vi "getPosition.vi"(6 "Delay between send and receive [ms]":i32=100, 8 "error in (no error)":errorcluster, 11 "Monochromator in":refnum<class "Monochromator.lvclass">) -> (0 "error out":errorcluster, 2 "wavelength":dbl, 3 "Monochromator out":refnum<class "Monochromator.lvclass">)   [LabVIEW 2023, in "horiba.lvlib" / "Monochromator.lvclass"]
doc: "Returns the wavelength value, in nm, of the monochromator's current position."
uses:
  Monochromator.lvclass
  d9b87029-586e-44ee-a6e5-d4a5e0edce38.vi
  b59fd1e7-dcda-425c-bd6c-61aafb79e7f4.vi
  GenericDevice/GenericDevice.lvclass
  WavelengthPosition.ctl
panel:
  # "Connector Pane"
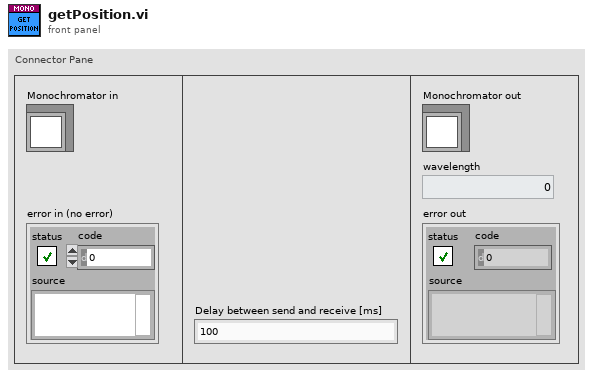
[diagram p1: front panel]
types:
  T1 = typedef "horiba.lvlib/Monochromator.lvclass/WavelengthPosition.ctl" = cluster{"wavelength":dbl}
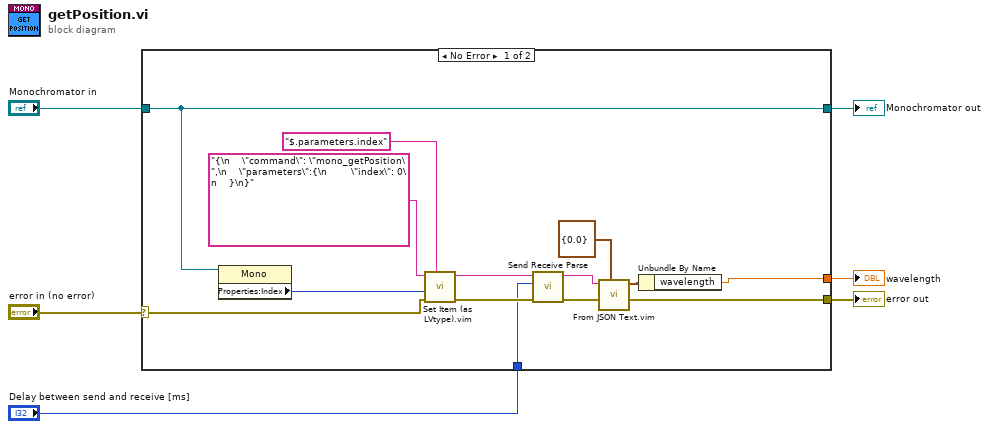
[diagram p0: block diagram]
diagram:
  n1 = case shown="No Error" "error in (no error)" {
    selector: "error in (no error)" -> [w16 w22]
    tunnel: [w15 w22] -> w5
    tunnel: [w18 w21] -> w3
    tunnel: "Monochromator in" -> [w18 w21]
    tunnel: [w8 _] -> w2
    tunnel: "Delay between send and receive [ms]" -> [w7 _]
    frame No Error {
      n2 = property class="Mono"(reference=w18) -> ("Properties:Index"=w17:i32)  [unwired: 1 in, 2 out]
      n3 = call "Set Item (as LVtype).vim"("$Path or Item Name"="$.parameters.index", "error in (no error)"=w16, "Anything"=w17, "JSON"="{\n    \"command\": \"mono_getPosition\",\n    \"parameters\":{\n        \"index\": 0\n    }\n}") -> ("error out"=w14:errorcluster, "<JSON>"=w11:string)  [unwired: 4 in, 1 out]
      n4 = call "Send Receive Parse.vi"("error in"=w14, "Delay between send and receive [ms]"=w7, "<JSON>"=w11) -> ("error out"=w12:errorcluster, "results-JSON string"=w13:string)  [unwired: 6 in, 1 out]
      n5 = call "From JSON Text.vim"("Data Type and Default Value"=T1 {"wavelength"=0.0} ("Position"), "error in (no error)"=w12, "JSON"=w13) -> ("error out"=w15:errorcluster, "Data out"=w10:T1)  [unwired: 7 in]
      n6 = Unbundle By Name(w10) -> ("wavelength"=w8:dbl)
    }
    frame Error {
    }
  }
  "error out" <- w5
  "Monochromator out" <- w3
  "wavelength" <- w2
